vi "CMD_TAN.vi"(6 "Gantry in":refnum<class "Gantry.lvclass">, 8 "error in (no error)":errorcluster, 10 "Arguments":string[](array[string]), 11 "gScript Interpreter in":refnum<class "gScript Interpreter.lvclass">) -> (0 "error out":errorcluster, 3 "gScript Interpreter out":refnum<class "gScript Interpreter.lvclass">, 4 "Gantry out":refnum<class "Gantry.lvclass">)   [LabVIEW 2023, in "gScript Interpreter.lvclass"]
uses:
  gScript Interpreter.lvclass
  Shared Components/Gantry Class/Gantry.lvclass
  Type Definitions/Memory Cell.ctl
  Type Definitions/Memory Cell Type Enum.ctl
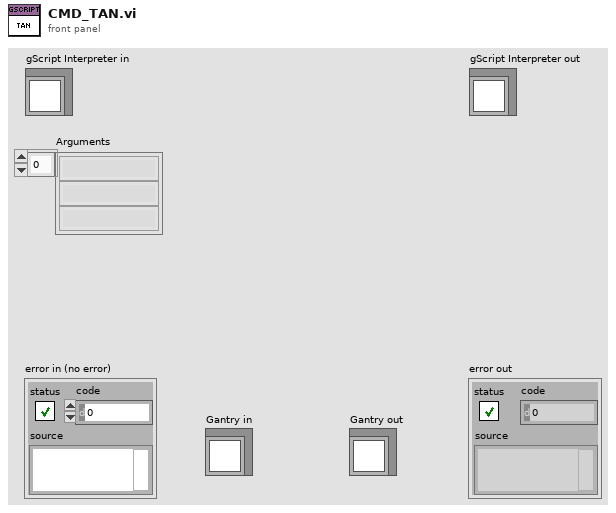
[diagram p1: front panel]
types:
  T1 = typedef "Memory Cell Type Enum.ctl" = enum16{"integer", "float", "vector", "rotation"}
  T2 = typedef "Memory Cell.ctl" = cluster{"type":T1, "x":dbl, "y":dbl, "z":dbl, "w":dbl}
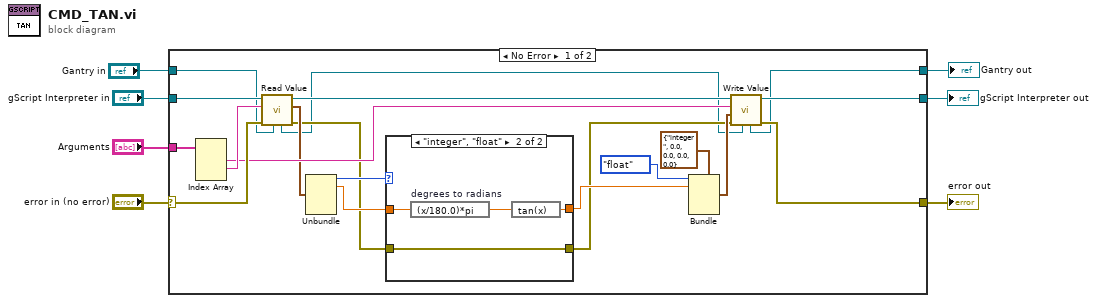
[diagram p0: block diagram]
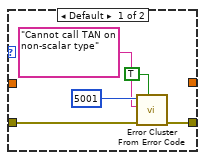
[diagram p2: hidden frame]
diagram:
  n1 = case shown="No Error" "error in (no error)" {
    selector: "error in (no error)" -> [w25 w39]
    tunnel: [w18 w39] -> w6
    tunnel: [w19 w38] -> w4
    tunnel: "gScript Interpreter in" -> [w26 w38]
    tunnel: "Arguments" -> [w27 _]
    tunnel: "Gantry in" -> [w10 w37]
    tunnel: [w8 w37] -> w1
    frame No Error {
      n2 = Index Array(array=w27) -> (element #1=w23:string, element #2=w24:string)  [unwired: 3 in, 1 out]
      n3 = call-dynamic "Read Value.vi"("Gantry in"=w10, "error in (no error)"=w25, "String in"=w24, "gScript Interpreter in"=w26) -> ("error out"=w12:errorcluster, "Memory Cell"=w22:T2, "gScript Interpreter out"=w17:refnum<class "gScript Interpreter.lvclass">, "Gantry out"=w9:refnum<class "Gantry.lvclass">)  [unwired: 4 in]
      n4 = Unbundle(w22) -> ("type"=w16:T1, "x"=w15:dbl)  [unwired: 3 out]
      n5 = case shown="\"integer\", \"float\"" w16 {
        tunnel: w15 -> [_ w34]
        tunnel: [_ w36] -> w14
        tunnel: w12 -> [w28 w35]
        tunnel: [w32 w35] -> w11
        frame Default {
          n6 = call <vilib>:"Error Cluster From Error Code.vi"("show call chain? (False)"=TRUE, "error in (no error)"=w28, "error message (\"\")"="Cannot call TAN on non-scalar type" ("error message (\"\")"), "error code (0)"=5001) -> ("error out"=w32:errorcluster)  [unwired: 5 in]
        }
        frame "integer", "float" {
          n7 = expression code="(x/180.0)*pi" "degrees to radians"(w34) -> (w33:dbl)
          n8 = expression code="tan(x)"(w33) -> (w36:dbl)
        }
      }
      n9 = Bundle(cluster=T2 {"type"=enum."integer", "x"=0.0, "y"=0.0, "z"=0.0, "w"=0.0} ("Memory Cell"), "type"=Memory_Cell_Type_Enum."float", "x"=w14) -> (w20:T2)  [unwired: 3 in]
      n10 = call-dynamic "Write Value.vi"("Gantry in"=w9, "error in (no error)"=w11, "Value"=w20, "Address"=w23, "gScript Interpreter in"=w17) -> ("error out"=w18:errorcluster, "gScript Interpreter out"=w19:refnum<class "gScript Interpreter.lvclass">, "Gantry out"=w8:refnum<class "Gantry.lvclass">)  [unwired: 4 in]
    }
    frame Error {
    }
  }
  "error out" <- w6
  "gScript Interpreter out" <- w4
  "Gantry out" <- w1
